vi "Read SubPnl Refnum.vi"(8 "error in (no error)":errorcluster, 11 "Show or Hide Quick Settings Msg in":refnum<class "Show or Hide Quick Settings Msg.lvclass">) -> (0 "error out":errorcluster, 2 "SubPnl Refnum":refnum<vi>, 3 "Show or Hide Quick Settings Msg out":refnum<class "Show or Hide Quick Settings Msg.lvclass">)   [LabVIEW 2014, in "HIJ Vision Display.lvlib" / "Show or Hide Quick Settings Msg.lvclass"]
uses:
  Show or Hide Quick Settings Msg.lvclass
  Show or Hide Quick Settings Msg.lvclass/Show or Hide Quick Settings Msg.ctl
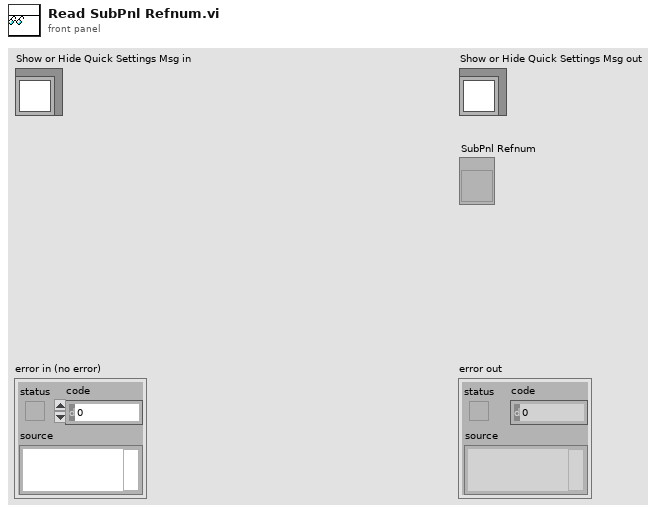
[diagram p1: front panel]
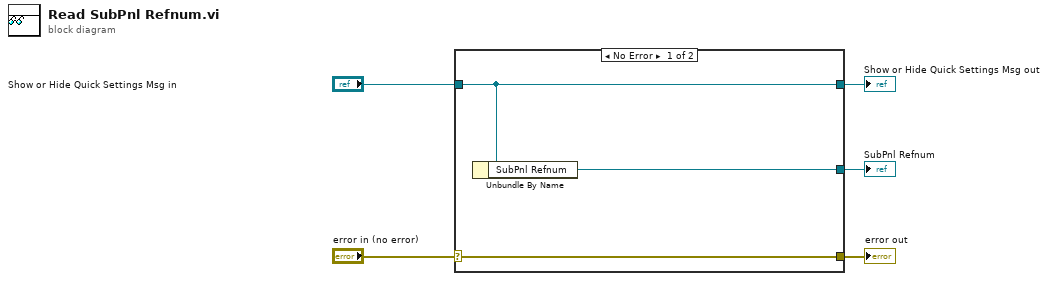
[diagram p0: block diagram]
diagram:
  n1 = case shown="No Error" "error in (no error)" {
    selector: "error in (no error)" -> [w8 w9]
    tunnel: [w8 w9] -> w4
    tunnel: [w7 w10] -> w2
    tunnel: "Show or Hide Quick Settings Msg in" -> [w7 w10]
    tunnel: [w6 _] -> w1
    frame No Error {
      n2 = Unbundle By Name(w7) -> ("SubPnl Refnum"=w6:refnum<vi>)
    }
    frame Error {
    }
  }
  "error out" <- w4
  "Show or Hide Quick Settings Msg out" <- w2
  "SubPnl Refnum" <- w1
